vi "MeasureRMS.vi"(7 "stop":bool, 8 "Samples":dbl, 9 "Sampling Rate":dbl) -> (0 "Error Out":errorcluster, 1 "Waveform Graph":dynamicdata(graph), 2 "RMS":dbl)   [LabVIEW 2015]
doc: "MeasureRMS that measures an analog signal from AI with given sampling rate and number of samples, and outputs a waveform and rms value for measured signal."
uses:
  <vilib>/Analysis/5stat.llb/RMS (DBL).vi
  <vilib>/Analysis/NI_AALPro.lvlib
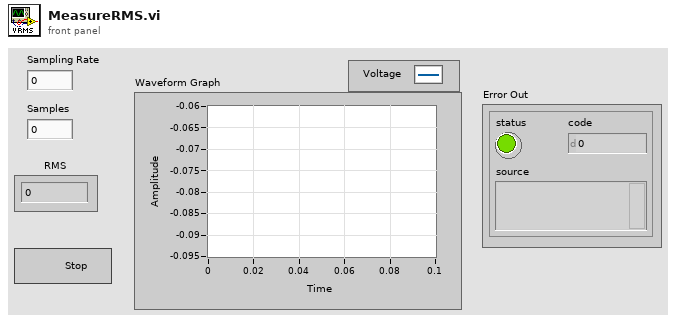
[diagram p1: front panel]
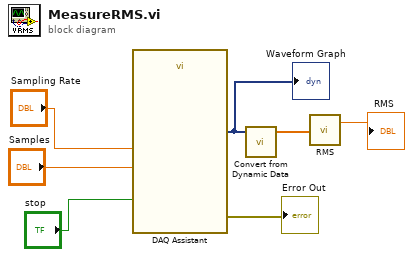
[diagram p0: block diagram]
diagram:
  n1 = call "DAQ Assistant"("rate"="Sampling Rate", "number of samples"="Samples", "stop (T)"="stop") -> ("data"=w3:dynamicdata, "error out"=→"Error Out":errorcluster)  [unwired: 14 in, 1 out]
  "Waveform Graph" <- w3
  n2 = call "Convert from Dynamic Data"("Dynamic Data Type"=w3) -> ("Array"=w2:dbl[])  [unwired: 3 in]
  n3 = call-poly <vilib>:"RMS.vi"("X"=w2) -> ("rms value"=→"RMS":dbl)  [unwired: 1 out]
